vi "SetM2VelocityPID.vi"(0 "VISA Refnum in":refnum<visa-resource-name>, 1 "Kd":u32 max=127 step=1, 2 "QPPS":u32 max=127 step=1, 5 "Ki":u32 max=127 step=1, 7 "Kp":u32 max=127 step=1, 9 "Address":u8, 11 "error in (no error)":errorcluster) -> (4 "VISA Refnum out":refnum<visa-resource-name>, 6 "Valid":bool, 15 "error out":errorcluster)   [LabVIEW 2015, in "Ion Motion Roboclaw.lvlib"]
uses:
  <instrlib>/Ion Motion Roboclaw/Ion Motion Roboclaw.lvlib
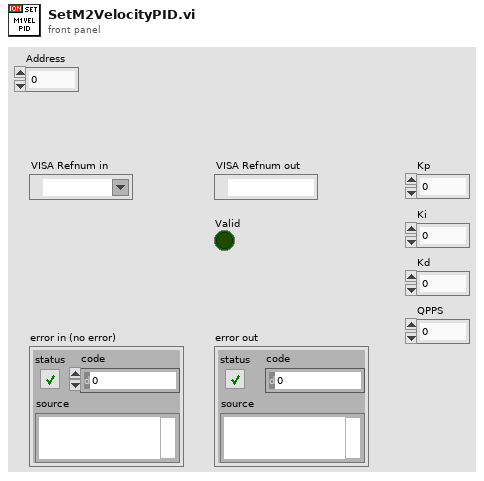
[diagram p1: front panel]
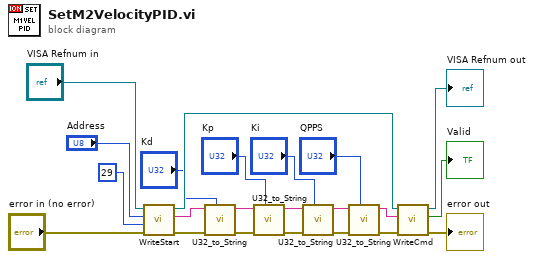
[diagram p0: block diagram]
diagram:
  n1 = call <instrlib>:"WriteStart.vi"("error in (no error)"="error in (no error)", "Cmd"=u8 29, "Address"="Address", "VISA Refnum in"="VISA Refnum in") -> ("error out"=w13:errorcluster, "String Out"=w11:string, "VISA Refnum out"=w21:refnum<visa-resource-name>)  [unwired: 5 in]
  n2 = call <instrlib>:"U32_to_String.vi"("number"="Kd", "error in (no error)"=w13, "String In"=w11) -> ("error out"=w14:errorcluster, "String Out"=w10:string)  [unwired: 5 in]
  n3 = call <instrlib>:"U32_to_String.vi"("number"="Kp", "error in (no error)"=w14, "String In"=w10) -> ("error out"=w15:errorcluster, "String Out"=w9:string)  [unwired: 5 in]
  n4 = call <instrlib>:"U32_to_String.vi"("number"="Ki", "error in (no error)"=w15, "String In"=w9) -> ("error out"=w16:errorcluster, "String Out"=w8:string)  [unwired: 5 in]
  n5 = call <instrlib>:"U32_to_String.vi"("number"="QPPS", "error in (no error)"=w16, "String In"=w8) -> ("error out"=w17:errorcluster, "String Out"=w7:string)  [unwired: 5 in]
  n6 = call <instrlib>:"WriteCmd.vi"("error in (no error)"=w17, "write buffer"=w7, "VISA Refnum in"=w21) -> ("error out"=→"error out":errorcluster, "Valid"=→"Valid":bool, "VISA Refnum out"=→"VISA Refnum out":refnum<visa-resource-name>)  [unwired: 2 in]
